vi "tdms_read.vi"() -> ()   [LabVIEW 2019]
panel:
  out "Signals":dynamicdata(graph)
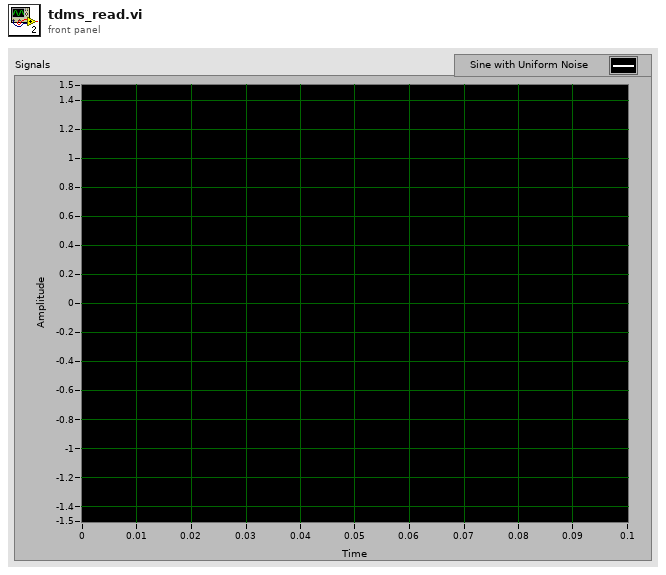
[diagram p1: front panel]
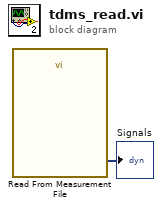
[diagram p0: block diagram]
diagram:
  n1 = call "Read From Measurement File"() -> ("Signals"=→"Signals":dynamicdata)  [unwired: 6 in, 5 out]
